vi "Timer FGV.vi"(7 "Action":T1, 8 "error in (no error)":errorcluster) -> (0 "error out":errorcluster, 3 "Elapsed Time":dbl)   [LabVIEW 2015]
uses:
  Timer Actions.ctl
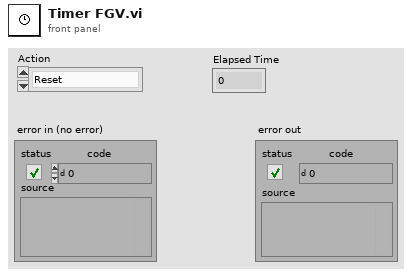
[diagram p1: front panel]
types:
  T1 = typedef "Timer Actions.ctl" = enum16{"Reset", "Get"}
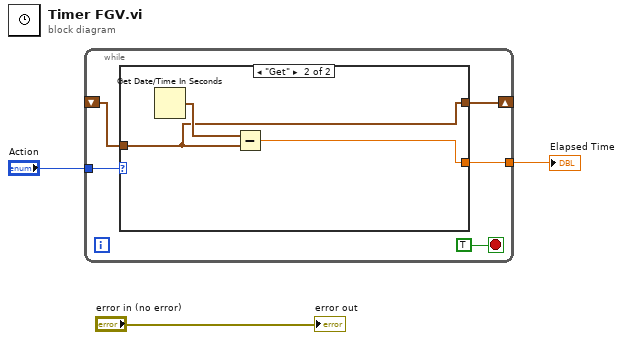
[diagram p0: block diagram]
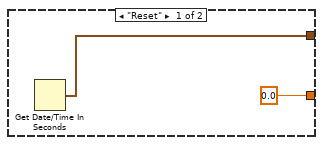
[diagram p2: hidden frame]
diagram:
  n1 = while {
    shift-right: [w6] -> _
    shift-left: _ -> [w4]
    tunnel: "Action" -> [w7]
    tunnel: [w5] -> w1
    stop <- TRUE stop-if-true
    n2 = case shown="\"Get\"" w7 {
      tunnel: [w10 w11] -> w6
      tunnel: [0.0 ("Elapsed Time") w12] -> w5
      tunnel: w4 -> [_ w11]
      frame "Reset" {
        n3 = Get Date/Time In Seconds() -> (seconds since 1Jan1904=w10:timestamp)
      }
      frame "Get" {
        n4 = Get Date/Time In Seconds() -> (seconds since 1Jan1904=w13:timestamp)
        n5 = Subtract(x=w13, y=w11) -> (x-y=w12:dbl)
      }
    }
  }
  "Elapsed Time" <- w1
  "error out" <- "error in (no error)"
